vi "Setup file output channels.vi"(5 "Stimulus":T2={"type"=enum."Zero", "sinfreq start"=0.0, "sinfreq end"=0.0, "sinamp start"=0.0, "sinamp end"=0.0, "noise freq lo"=0.0, "noise freq hi"=0.0, "noiseamp start"=0.0, "noiseamp end"=0.0, "stimdur"=0.0, "before dur"=0.0, "after dur"=0.0, "pulse data"={"time"=[], "phase/vel"=[], "dir/shift"=[], "amplitude"=[], "duration"=[]}} {"noise freq hi" min=0.0 step=0.5; "noise freq lo" min=0.0 step=0.5; "noiseamp end" min=0.0 step=0.5; "noiseamp start" min=0.0 step=0.5}, 7 "motor":dbl[](array[numeric]), 8 "error in":errorcluster, 9 "Sampling data":T5={"Channels"=[], "Sampling freq"=0.0, "Output freq"=0.0, "Update freq"=0.0, "Steps per rev"=0, "Counts per rev"=0, "Amplifier"="", "Motor driver"="", "Step bit"=0, "Max speed"=0.0, "Max accel"=0.0, "Pos gain"=0.0, "Vel gain"=0.0, "counter"="Dev1/ctr0"} {"Channels"."Hi cutoff" items=["500"=500.0, "1k"=1000.0, "5k"=5000.0, "10k"=10000.0, "20k"=20000.0]; "Channels"."Lo cutoff" items=["0.1"=0.1, "1"=1.0, "10"=10.0, "100"=100.0, "300"=300.0]; "Channels"."Gain" items=["x100"=100, "x1000"=1000, "x10000"=10000]}, 10 "stimphases in":T1, 11 "file ref in":T7 format="%.0x") -> (0 "error out":errorcluster, 1 "Sampling data out":T5={"Channels"=[], "Sampling freq"=0.0, "Output freq"=0.0, "Update freq"=0.0, "Steps per rev"=0, "Counts per rev"=0, "Amplifier"="", "Motor driver"="", "Step bit"=0, "Max speed"=0.0, "Max accel"=0.0, "Pos gain"=0.0, "Vel gain"=0.0, "counter"="Dev1/ctr0"} {"Channels"."Hi cutoff" items=["500"=500.0, "1k"=1000.0, "5k"=5000.0, "10k"=10000.0, "20k"=20000.0]; "Channels"."Lo cutoff" items=["0.1"=0.1, "1"=1.0, "10"=10.0, "100"=100.0, "300"=300.0]; "Channels"."Gain" items=["x100"=100, "x1000"=1000, "x10000"=10000]}, 2 "dset ref":i32, 3 "file ref out":T7 format="%.0x")   [LabVIEW 2013]
uses:
  <vilib>/addons/h5labview2/base/hid_t.ctl
  Sampling info.ctl
  Channel.ctl
  Stimulus.ctl
  Stimulus type.ctl
  Pulse data.ctl
  Stim phases.ctl
  <vilib>/addons/h5labview2/base/lib_path.vi
  <vilib>/addons/h5labview2/base/H5Equery.vi
  <vilib>/addons/h5labview2/attrib/H5Awrite.llb/H5Awrite.xnode
  <vilib>/addons/h5labview2/dataset/H5Dwrite.llb/H5Dwrite.xnode
  <vilib>/addons/h5labview2/group/H5G.lvlib
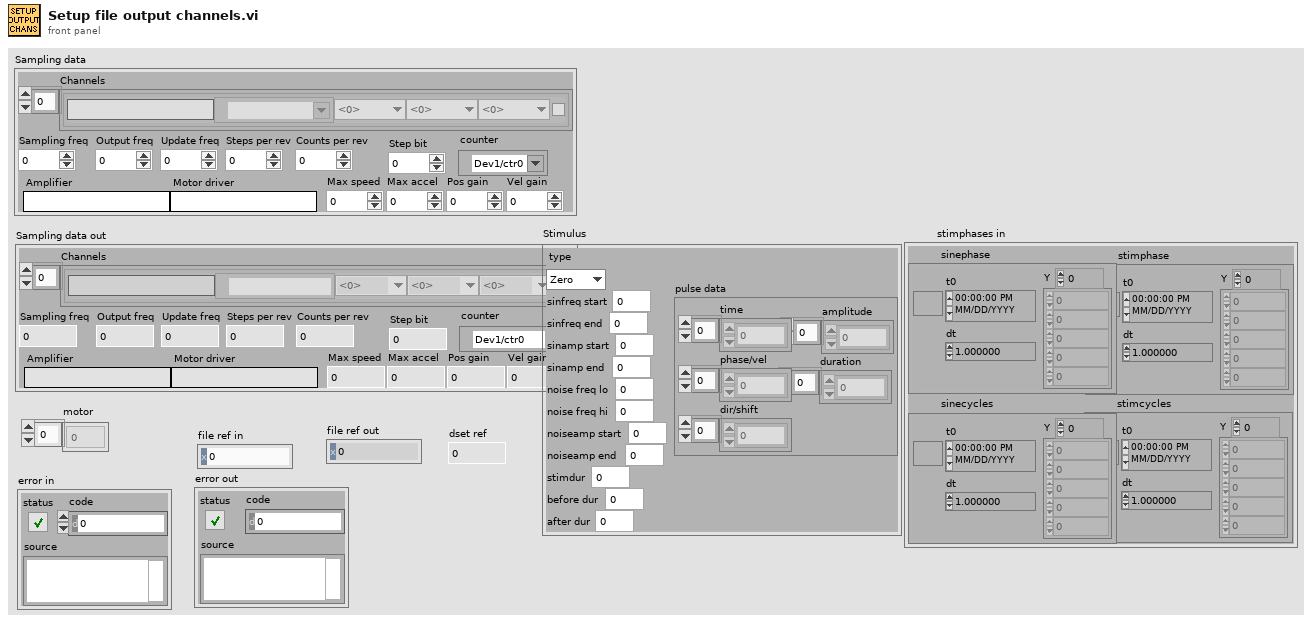
[diagram p1: front panel]
types:
  T1 = typedef "Stim phases.ctl" = cluster{"sinephase":waveform(dbl), "sinecycles":waveform(dbl), "stimphase":waveform(dbl), "stimcycles":waveform(dbl)}
  T2 = typedef "Stimulus.ctl" = cluster{"type":T3, "sinfreq start":dbl, "sinfreq end":dbl, "sinamp start":dbl, "sinamp end":dbl, "noise freq lo":dbl, "noise freq hi":dbl, "noiseamp start":dbl, "noiseamp end":dbl, "stimdur":dbl, "before dur":dbl, "after dur":dbl, "pulse data":T4}
  T3 = typedef "Stimulus type.ctl" = enum16{"Sine", "Zero", "Frequency sweep", "Two frequency", "Amplitude sweep", "Pulses", "Shifts", "Ramps"}
  T4 = typedef "Pulse data.ctl" = cluster{"time":dbl[], "phase/vel":dbl[], "dir/shift":dbl[], "amplitude":dbl[], "duration":dbl[]}
  T5 = typedef "Sampling info.ctl" = cluster{"Channels":T6[], "Sampling freq":dbl, "Output freq":dbl, "Update freq":dbl, "Steps per rev":i32, "Counts per rev":i32, "Amplifier":string, "Motor driver":string, "Step bit":u8, "Max speed":dbl, "Max accel":dbl, "Pos gain":dbl, "Vel gain":dbl, "counter":tag}
  T6 = typedef "Channel.ctl" = cluster{"Name":string, "Chan":tag, "Gain":u32, "Lo cutoff":dbl, "Hi cutoff":dbl, "Notch":bool}
  T7 = typedef "hid_t.ctl" = i32
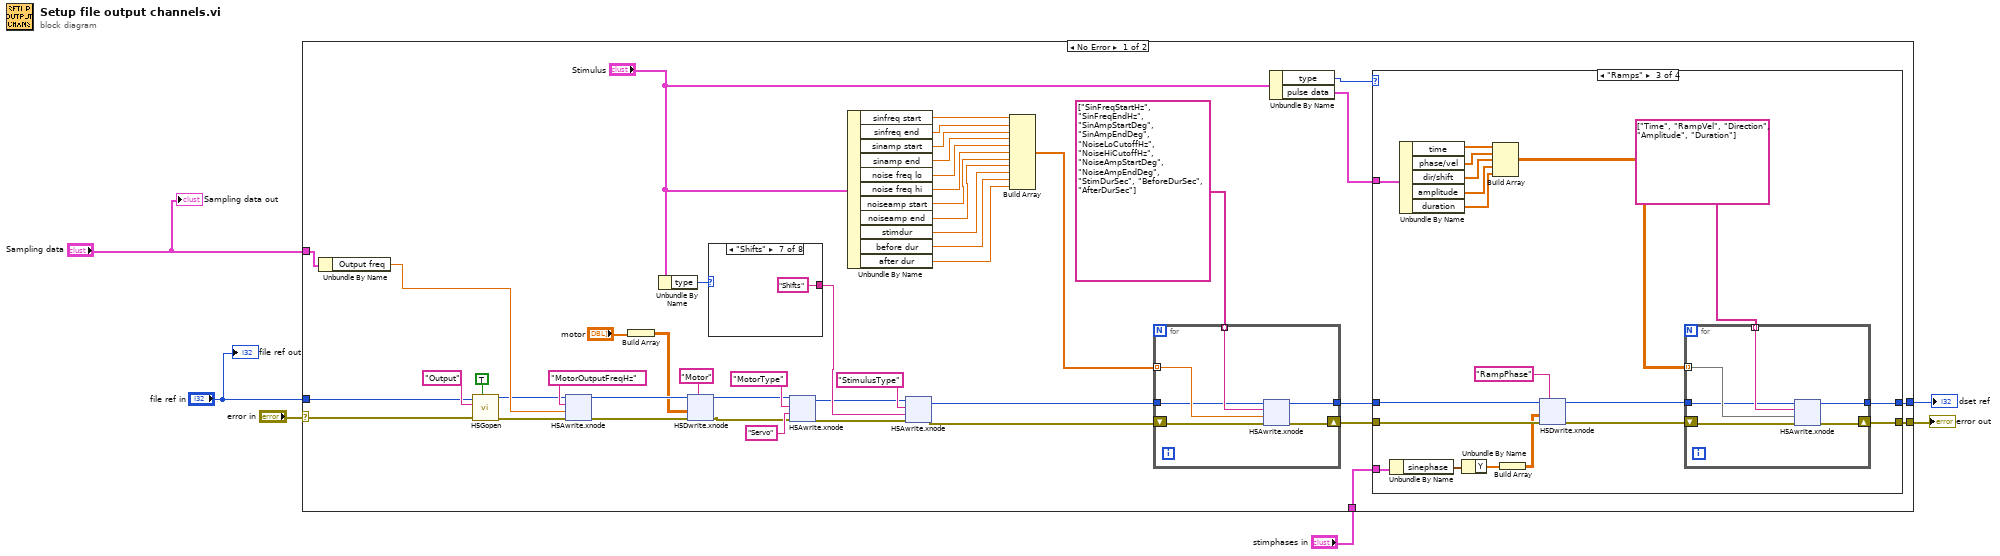
[diagram p0: block diagram]
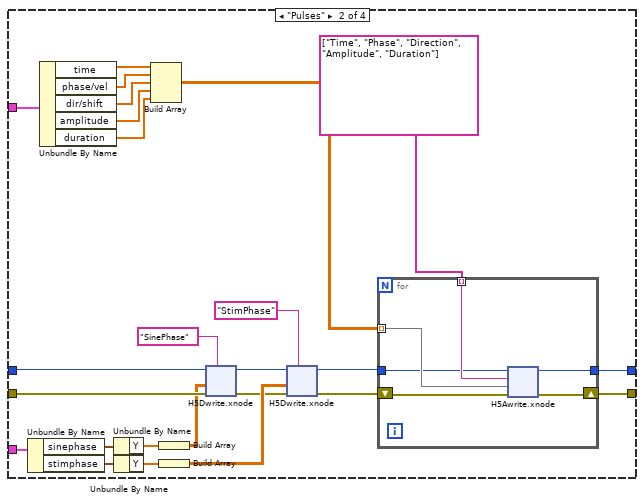
[diagram p3: hidden frame]
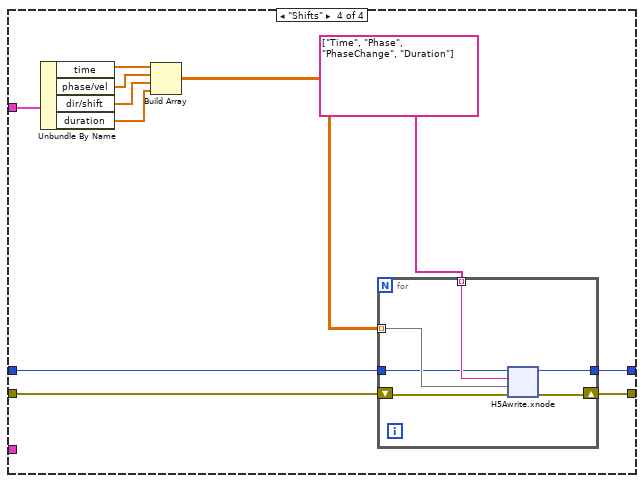
[diagram p4: hidden frame]
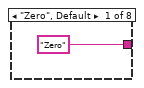
[diagram p5: hidden frame]
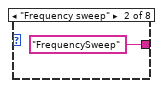
[diagram p6: hidden frame]
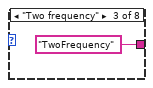
[diagram p7: hidden frame]
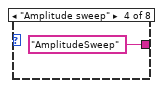
[diagram p8: hidden frame]
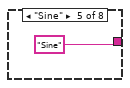
[diagram p9: hidden frame]
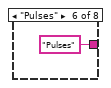
[diagram p10: hidden frame]
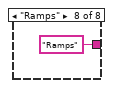
[diagram p11: hidden frame]
diagram:
  n1 = case shown="No Error" "error in" {
    selector: "error in" -> [w49 w340]
    tunnel: [w9 w340] -> w6
    tunnel: "file ref in" -> [w48 _]
    tunnel: "Sampling data" -> [w52 _]
    tunnel: [w11 _] -> w2
    tunnel: "stimphases in" -> [w7 _]
    frame No Error {
      n2 = Unbundle By Name(w52) -> ("Output freq"=w46:dbl)
      n3 = call <vilib>:"H5Gopen.vi"("create? (F)"=TRUE, "error in (no error)"=w49, "name"="Output", "ref in"=w48) -> ("error out"=w44:errorcluster, "group out"=w45:T7)  [unwired: 3 in]
      n4 = xnode "H5Awrite.xnode"("error in (no error)"=w44, "data"=w46, "attrib name"="MotorOutputFreqHz", "ref in"=w45) -> ("error out"=w39:errorcluster, "ref out"=w41:T7)  [unwired: 3 in, 1 out]
      n5 = Build Array("motor") -> (w16:dbl[][])
      n6 = Unbundle By Name("Stimulus") -> ("type"=w36:T3)
      n7 = xnode "H5Dwrite.xnode"("dataset name"="Motor", "error in (no error)"=w39, "data"=w16, "ref in"=w41) -> ("error out"=w38:errorcluster, "ref out"=w15:T7)  [unwired: 3 in, 1 out]
      n8 = case shown="\"Shifts\"" w36 {
        tunnel: ["Zero" ("attrib name") "FrequencySweep" ("attrib name") "TwoFrequency" ("attrib name") "AmplitudeSweep" ("attrib name") "Sine" ("attrib name") "Pulses" ("attrib name") "Shifts" ("attrib name") "Ramps" ("attrib name")] -> w35
        frame "Zero", Default {
        }
        frame "Frequency sweep" {
        }
        frame "Two frequency" {
        }
        frame "Amplitude sweep" {
        }
        frame "Sine" {
        }
        frame "Pulses" {
        }
        frame "Shifts" {
        }
        frame "Ramps" {
        }
      }
      n9 = xnode "H5Awrite.xnode"("error in (no error)"=w38, "data"="Servo" ("attrib name"), "attrib name"="MotorType", "ref in"=w15) -> ("error out"=w34:errorcluster, "ref out"=w33:T7)  [unwired: 3 in, 1 out]
      n10 = Unbundle By Name("Stimulus") -> ("sinfreq start"=w32:dbl, "sinfreq end"=w31:dbl, "sinamp start"=w30:dbl, "sinamp end"=w29:dbl, "noise freq lo"=w28:dbl, "noise freq hi"=w27:dbl, "noiseamp start"=w26:dbl, "noiseamp end"=w25:dbl, "stimdur"=w24:dbl, "before dur"=w23:dbl, "after dur"=w22:dbl)
      n11 = xnode "H5Awrite.xnode"("error in (no error)"=w34, "data"=w35, "attrib name"="StimulusType", "ref in"=w33) -> ("error out"=w19:errorcluster, "ref out"=w18:T7)  [unwired: 3 in, 1 out]
      n12 = Build Array(w32, w31, w30, w29, w28, w27, w26, w25, w24, w23, w22) -> (w21:dbl[])
      n13 = for {
        tunnel: w21 -> [w240] mode=indexing
        tunnel: string[] ["SinFreqStartHz", "SinFreqEndHz", "SinAmpStartDeg", "SinAmpEndDeg", "NoiseLoCutoffHz", "NoiseHiCutoffHz", "NoiseAmpStartDeg", "NoiseAmpEndDeg", "StimDurSec", "BeforeDurSec", "AfterDurSec"] -> [w241] mode=indexing
        tunnel: w18 -> [w238]
        tunnel: [w237] -> w12
        shift-right: [w236] -> w10
        shift-left: w19 -> [w239]
        n14 = xnode "H5Awrite.xnode"("error in (no error)"=w239, "data"=w240, "attrib name"=w241, "ref in"=w238) -> ("error out"=w236:errorcluster, "ref out"=w237:T7)  [unwired: 3 in, 1 out]
      }
      n15 = Unbundle By Name("Stimulus") -> ("type"=w13:T3, "pulse data"=w8:T4)
      n16 = case shown="\"Ramps\"" w13 {
        tunnel: w12 -> [w54 w68 w147 w204]
        tunnel: [w54 w71 w150 w202] -> w11
        tunnel: w10 -> [w53 w67 w146 w203]
        tunnel: [w53 w70 w149 w201] -> w9
        tunnel: w8 -> [_ w79 w158 w211]
        tunnel: w7 -> [_ w66 w145 _]
        frame "Zero", Default {
        }
        frame "Pulses" {
          n17 = Unbundle By Name(w66) -> ("sinephase"=w65:waveform(dbl), "stimphase"=w62:waveform(dbl))
          n18 = Unbundle By Name(w79) -> ("time"=w78:dbl[], "phase/vel"=w77:dbl[], "dir/shift"=w76:dbl[], "amplitude"=w75:dbl[], "duration"=w74:dbl[])
          n19 = Unbundle By Name(w65) -> ("Y"=w64:dbl[])
          n20 = Unbundle By Name(w62) -> ("Y"=w61:dbl[])
          n21 = Build Array(w78, w77, w76, w75, w74) -> (w72:dbl[][])
          n22 = Build Array(w64) -> (w60:dbl[][])
          n23 = Build Array(w61) -> (w59:dbl[][])
          n24 = xnode "H5Dwrite.xnode"("dataset name"="SinePhase", "error in (no error)"=w67, "data"=w60, "ref in"=w68) -> ("error out"=w57:errorcluster, "ref out"=w58:T7)  [unwired: 3 in, 1 out]
          n25 = xnode "H5Dwrite.xnode"("dataset name"="StimPhase", "error in (no error)"=w57, "data"=w59, "ref in"=w58) -> ("error out"=w55:errorcluster, "ref out"=w56:T7)  [unwired: 3 in, 1 out]
          n26 = for {
            tunnel: w72 -> [w120] mode=indexing
            tunnel: string[] ["Time", "Phase", "Direction", "Amplitude", "Duration"] -> [w121] mode=indexing
            tunnel: w56 -> [w118]
            tunnel: [w117] -> w71
            shift-right: [w116] -> w70
            shift-left: w55 -> [w119]
            n27 = xnode "H5Awrite.xnode"("error in (no error)"=w119, "data"=w120, "attrib name"=w121, "ref in"=w118) -> ("error out"=w116:errorcluster, "ref out"=w117:T7)  [unwired: 3 in, 1 out]
          }
        }
        frame "Ramps" {
          n28 = Unbundle By Name(w145) -> ("sinephase"=w144:waveform(dbl))
          n29 = Unbundle By Name(w158) -> ("time"=w157:dbl[], "phase/vel"=w156:dbl[], "dir/shift"=w155:dbl[], "amplitude"=w154:dbl[], "duration"=w153:dbl[])
          n30 = Unbundle By Name(w144) -> ("Y"=w143:dbl[])
          n31 = Build Array(w157, w156, w155, w154, w153) -> (w151:dbl[][])
          n32 = Build Array(w143) -> (w142:dbl[][])
          n33 = xnode "H5Dwrite.xnode"("dataset name"="RampPhase", "error in (no error)"=w146, "data"=w142, "ref in"=w147) -> ("error out"=w140:errorcluster, "ref out"=w141:T7)  [unwired: 3 in, 1 out]
          n34 = for {
            tunnel: w151 -> [w181] mode=indexing
            tunnel: string[] ["Time", "RampVel", "Direction", "Amplitude", "Duration"] -> [w182] mode=indexing
            tunnel: w141 -> [w179]
            tunnel: [w178] -> w150
            shift-right: [w177] -> w149
            shift-left: w140 -> [w180]
            n35 = xnode "H5Awrite.xnode"("error in (no error)"=w180, "data"=w181, "attrib name"=w182, "ref in"=w179) -> ("error out"=w177:errorcluster, "ref out"=w178:T7)  [unwired: 3 in, 1 out]
          }
        }
        frame "Shifts" {
          n36 = Unbundle By Name(w211) -> ("time"=w210:dbl[], "phase/vel"=w209:dbl[], "dir/shift"=w208:dbl[], "duration"=w207:dbl[])
          n37 = Build Array(w210, w209, w208, w207) -> (w205:dbl[][])
          n38 = for {
            tunnel: w205 -> [w216] mode=indexing
            tunnel: string[] ["Time", "Phase", "PhaseChange", "Duration"] -> [w217] mode=indexing
            tunnel: w204 -> [w214]
            tunnel: [w213] -> w202
            shift-right: [w212] -> w201
            shift-left: w203 -> [w215]
            n39 = xnode "H5Awrite.xnode"("error in (no error)"=w215, "data"=w216, "attrib name"=w217, "ref in"=w214) -> ("error out"=w212:errorcluster, "ref out"=w213:T7)  [unwired: 3 in, 1 out]
          }
        }
      }
    }
    frame Error {
    }
  }
  "dset ref" <- w2
  "error out" <- w6
  "file ref out" <- "file ref in"
  "Sampling data out" <- "Sampling data"
